vi "New Major Frame.vi"(6 "loopCountSpecified (F)":bool, 8 "error in":errorcluster, 9 "loopCount (0: continous)":i32, 10 "Minor Frames":refnum<k24>[](array[refnum]), 11 "name":string) -> (0 "error out":errorcluster, 1 "Major Frame ID out":i32, 3 "new major frame":refnum<k24>)   [LabVIEW 2020, in "Ballard_1553_Hardware_ni.lvlib"]
uses:
  Ballard_1553_Hardware_ni.lvlib
  C:/Users/Administrator/Desktop/GIT/Ballard-MIL-STD-1553-Custom-Device/Source/System Explorer/SubVIs/Parse XML Ballard/1.2/BTIXML_SerDes.dll
  Ballard-MIL-STD-1553-Custom-Device/Source/System Explorer/SubVIs/Parse XML Ballard/1.2/BTIXML_SerDes.dll
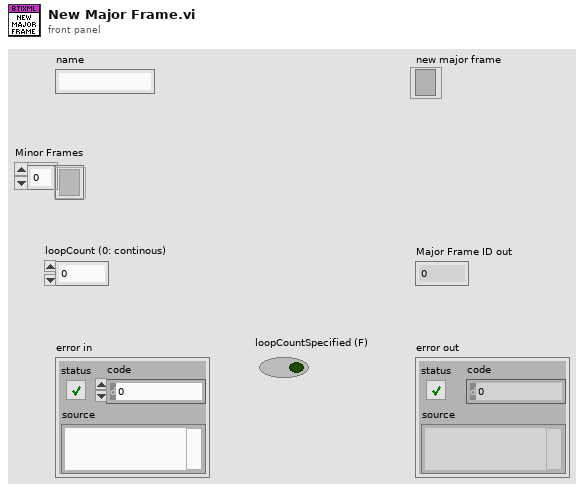
[diagram p1: front panel]
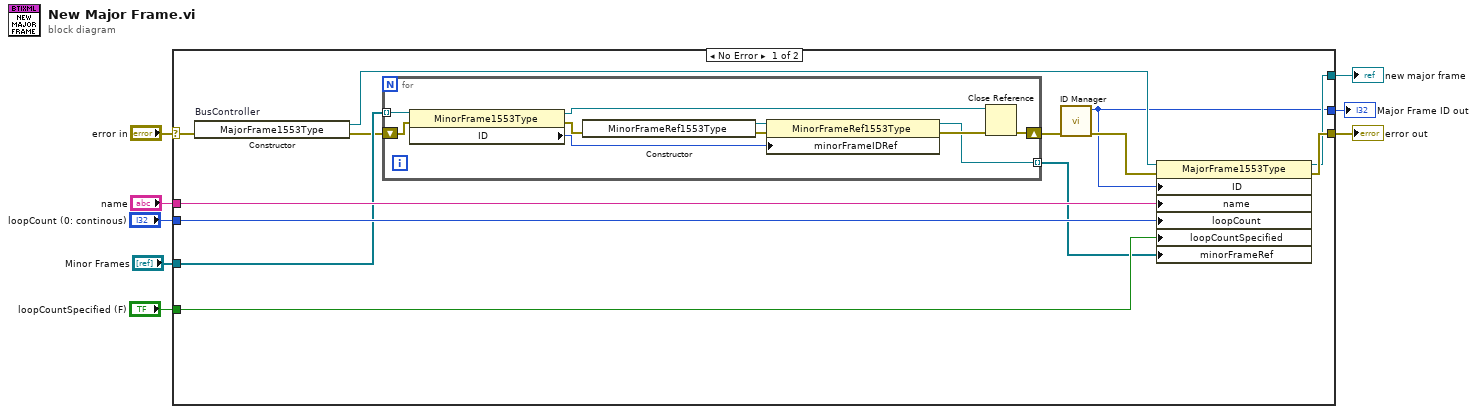
[diagram p0: block diagram]
diagram:
  n1 = case shown="No Error" "error in" {
    selector: "error in" -> [w21 w32]
    tunnel: [w20 w32] -> w7
    tunnel: [w19 _] -> w4
    tunnel: "name" -> [w16 _]
    tunnel: "Minor Frames" -> [w13 _]
    tunnel: "loopCountSpecified (F)" -> [w15 _]
    tunnel: "loopCount (0: continous)" -> [w14 _]
    tunnel: [w9 _] -> w1
    frame No Error {
      n2 = constructor on="BusController" class="MajorFrame1553Type"(error in=w21) -> (reference out=w18:refnum<k24>, error out=w12:errorcluster)  [unwired: 2 in, 1 out]
      n3 = for {
        tunnel: w13 -> [w31] mode=indexing
        shift-right: [w27] -> w11
        shift-left: w12 -> [w30]
        tunnel: [w22] -> w10 mode=indexing
        n4 = property class="MinorFrame1553Type"(reference=w31, error in=w30) -> (reference out=w28:refnum<k24>, error out=w29:errorcluster, "ID"=w23:i32)
        n5 = constructor class="MinorFrameRef1553Type"(error in=w29) -> (reference out=w24:refnum<k24>, error out=w26:errorcluster)  [unwired: 2 in, 1 out]
        n6 = property class="MinorFrameRef1553Type"(reference=w24, error in=w26, "minorFrameIDRef"=w23) -> (reference out=w22:refnum<k24>, error out=w25:errorcluster)
        n7 = Close Reference(reference=w28, error in (no error)=w25) -> (error out=w27:errorcluster)
      }
      n8 = call "ID Manager.vi"("error in"=w11) -> ("error out"=w17:errorcluster, "ID out"=w9:i32)  [unwired: 9 in]
      n9 = property class="MajorFrame1553Type"(reference=w18, error in=w17, "ID"=w9, "name"=w16, "loopCount"=w14, "loopCountSpecified"=w15, "minorFrameRef"=w10) -> (reference out=w19:refnum<k24>, error out=w20:errorcluster)
    }
    frame Error {
    }
  }
  "error out" <- w7
  "new major frame" <- w4
  "Major Frame ID out" <- w1
